vi "Update User Input.vi"(8 "error in (no error)":errorcluster, 9 "Value":string, 10 "Key Focus":bool, 11 "User Input Reference":refnum<vi>) -> (0 "error out":errorcluster)   [LabVIEW 2020]
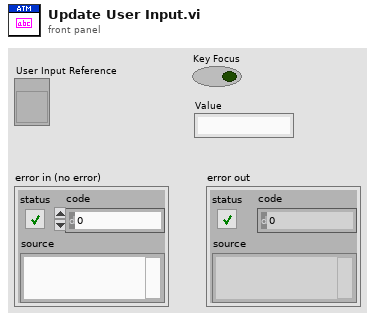
[diagram p1: front panel]
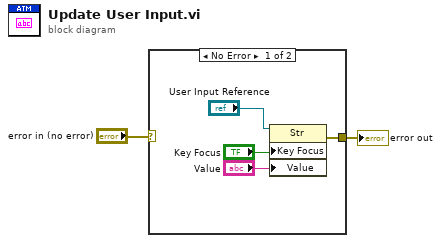
[diagram p0: block diagram]
diagram:
  n1 = case shown="No Error" "error in (no error)" {
    selector: "error in (no error)" -> [_ w7]
    tunnel: [w6 w7] -> w2
    frame No Error {
      n2 = property class="Str"(reference="User Input Reference", "Key Focus"="Key Focus", "Value"="Value") -> (error out=w6:errorcluster)  [unwired: 1 in, 1 out]
    }
    frame Error {
    }
  }
  "error out" <- w2
